vi "gpanel_close_galvos.vi"(8 "error in (no error)":errorcluster, 11 "galvo_panel in":refnum<class "galvo_panel.lvclass">) -> (0 "error out":errorcluster, 3 "galvo_panel out":refnum<class "galvo_panel.lvclass">)   [LabVIEW 2015, in "galvo_panel.lvclass"]
uses:
  galvo_panel.lvclass
  Hardware Class/hardware/hardware.lvclass
  UI/panel_class/panel.lvclass
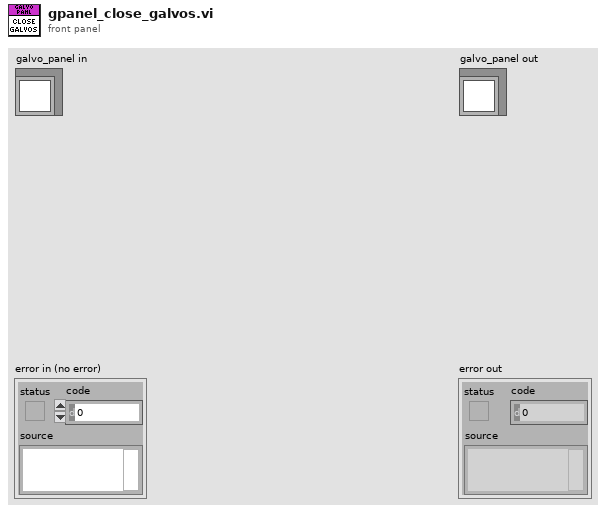
[diagram p1: front panel]
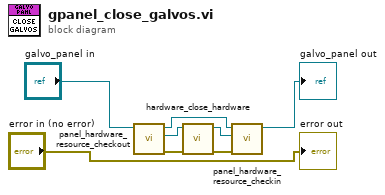
[diagram p0: block diagram]
diagram:
  n1 = call "panel_hardware_resource_checkout.vi"("panel in"="galvo_panel in") -> ("error out"=w5:errorcluster, "hardware.lvclass"=w6:refnum<class "hardware.lvclass">, "panel out"=w4:refnum<class "galvo_panel.lvclass">)  [unwired: 7 in, 1 out]
  n2 = call-dynamic "hardware_close_hardware.vi"("error in (no error)"=w5, "hardware in"=w6) -> ("error out"=w2:errorcluster, "hardware out"=w3:refnum<class "hardware.lvclass">)  [unwired: 8 in]
  n3 = call "panel_hardware_resource_checkin.vi"("error in (no error)"=w2, "hardware.lvclass"=w3, "panel in"=w4) -> ("panel out"=→"galvo_panel out":refnum<class "galvo_panel.lvclass">)  [unwired: 7 in, 1 out]
  "error out" <- "error in (no error)"
